vi "Enable_All.vi"(8 "error in (no error)":errorcluster, 11 "IB_Tree in":refnum<class "IB_Tree.lvclass">) -> (0 "error out":errorcluster, 3 "IB_Tree out":refnum<class "IB_Tree.lvclass">)   [LabVIEW 2020, in "IB_Tree.lvclass"]
uses:
  <vilib>/AppBuilder/IB_Classes/Tree/IB_Tree.lvclass
  <vilib>/AppBuilder/IB_Classes/Tree/IB_Tree.lvclass/IB_Tree.ctl
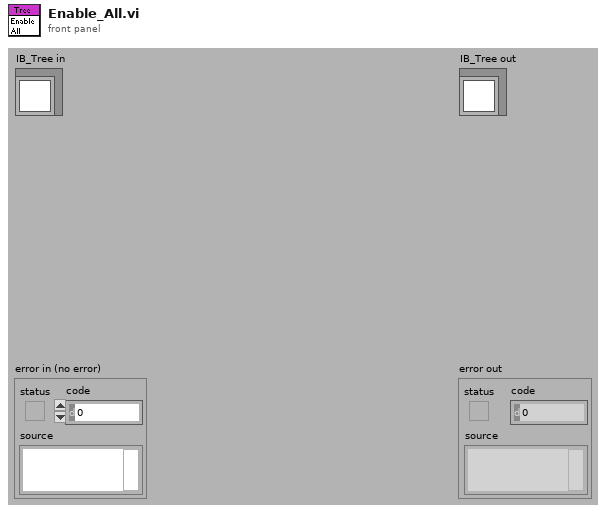
[diagram p1: front panel]
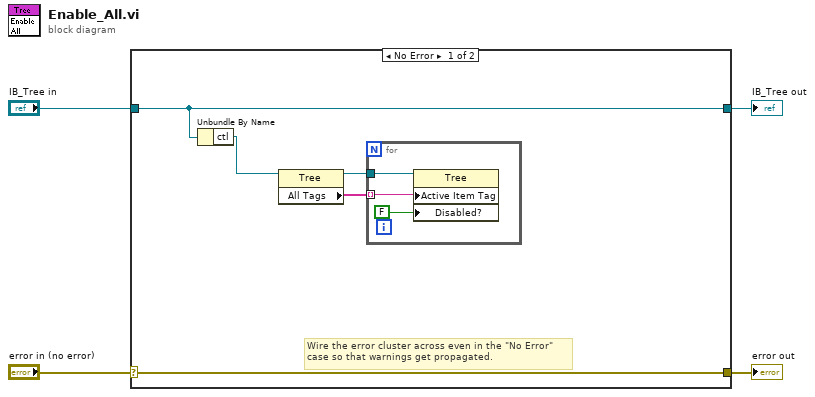
[diagram p0: block diagram]
diagram:
  n1 = case shown="No Error" "error in (no error)" {
    selector: "error in (no error)" -> [w9 w14]
    tunnel: [w9 w14] -> w3
    tunnel: [w8 w13] -> w1
    tunnel: "IB_Tree in" -> [w8 w13]
    frame No Error {
      # "Wire the error cluster across even in the \"No Error\"\ncase so that warnings get propagated."
      n2 = Unbundle By Name(w8) -> ("ctl"=w7:refnum<vi>)
      n3 = property class="Tree"(reference=w7) -> (reference out=w6:refnum<vi>, "All Tags"=w5:string[])  [unwired: 1 in, 1 out]
      n4 = for {
        tunnel: w6 -> [w12]
        tunnel: w5 -> [w10] mode=indexing
        n5 = property class="Tree"(reference=w12, "Active Item Tag"=w10, "Disabled?"=FALSE ("Active Item:Disabled?")) -> ()  [unwired: 1 in, 2 out]
      }
    }
    frame Error {
    }
  }
  "error out" <- w3
  "IB_Tree out" <- w1
